vi "Append a Page Break.vi"(8 "error in (no error)":errorcluster, 11 "xwpfParagraph in":refnum<class "xwpfParagraph.lvclass">) -> (0 "error out":errorcluster, 3 "xwpfParagraph out":refnum<class "xwpfParagraph.lvclass">)   [LabVIEW 2017, in "Word_Specific.lvlib" / "xwpfParagraph.lvclass"]
uses:
  xwpfParagraph.lvclass
  xwpfRun.PageBreak/xwpfRun.PageBreak.lvclass
  C:/Users/Neo/Desktop/Dev_Tools_BR/LabVIEW_NPOI/src/LabVIEW NPOI/xwpfRun/xwpfRun.lvclass
  xwpfParagraph.lvclass/xwpfParagraph.ctl
  C:/Users/Neo/Desktop/Dev_Tools_BR/LabVIEW_NPOI/src/lib/NPOI 2.1.1/NPOI.OOXML.dll
  lib/NPOI 2.1.1/NPOI.OOXML.dll
  xwpfRun/xwpfRun.lvclass
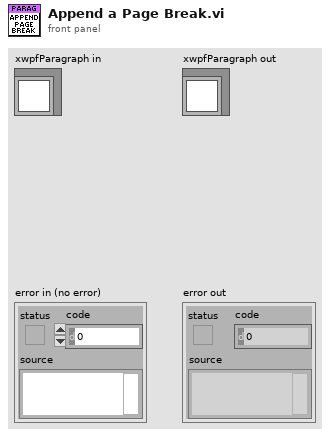
[diagram p1: front panel]
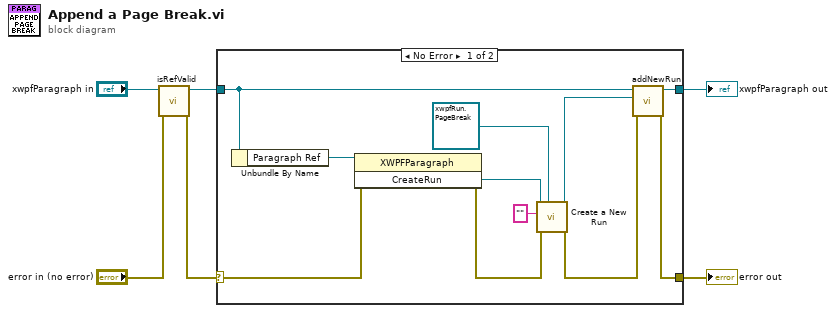
[diagram p0: block diagram]
diagram:
  n1 = call-dynamic "isRefValid.vi"("error in (no error)"="error in (no error)", "xwpfParagraph in"="xwpfParagraph in") -> ("error out"=w1:errorcluster, "xwpfParagraph out"=w3:refnum<class "xwpfParagraph.lvclass">)  [unwired: 8 in]
  n2 = case shown="No Error" w1 {
    selector: w1 -> [w9 w19]
    tunnel: [w11 w19] -> w6
    tunnel: [w14 w18] -> w4
    tunnel: w3 -> [w10 w18]
    frame No Error {
      n3 = Unbundle By Name(w10) -> ("Paragraph Ref"=w17:refnum<k24>)
      n4 = invoke class="XWPFParagraph" method="CreateRun"(reference=w17, error in=w9) -> (error out=w15:errorcluster, "CreateRun"=w16:refnum<k24>)  [unwired: 1 in, 1 out]
      n5 = call "Create a New Run.vi"("xwpfRun Type"=refnum<class "xwpfRun.PageBreak.lvclass"> refnum ("LabVIEW NPOI.lvlib:xwpfRun.PageBreak.lvclass"), "error in (no error)"=w15, "Text"="", "Run Ref"=w16) -> ("error out"=w12:errorcluster, "xwpfRun out"=w13:refnum<class "xwpfRun.PageBreak.lvclass">)  [unwired: 6 in]
      n6 = call "addNewRun.vi"("error in (no error)"=w12, "New Run"=w13, "xwpfParagraph in"=w10) -> ("error out"=w11:errorcluster, "xwpfParagraph out"=w14:refnum<class "xwpfParagraph.lvclass">)  [unwired: 7 in]
    }
    frame Error {
    }
  }
  "error out" <- w6
  "xwpfParagraph out" <- w4
